vi "init Tests.vi"(8 "error in (no error)":errorcluster caption="Error in", 11 "DeviceInterface Eingang":refnum<class "DeviceInterface.lvclass"> caption="DNL_LabVIEW Object in") -> (0 "error out":errorcluster caption="Error out", 3 "DeviceInterface Ausgang":refnum<class "DeviceInterface.lvclass"> caption="DNL_LabVIEW Object out")   [LabVIEW 2013, in "DeviceInterface.lvclass"]
doc: "Initilisiert die Standard-Tests für das Entsprechende Gerät"
uses:
  DeviceInterface.lvclass
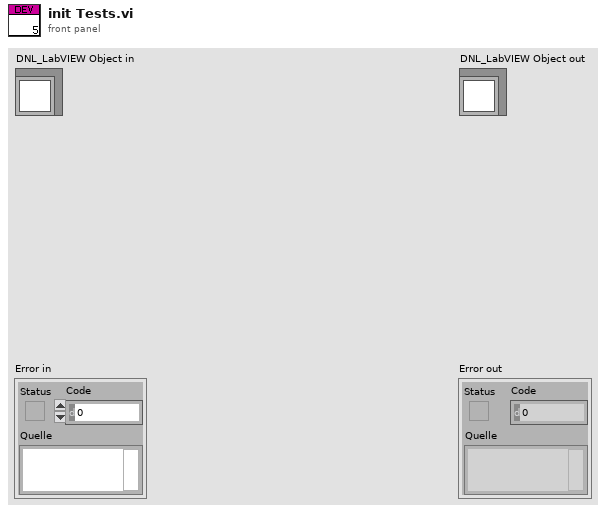
[diagram p1: front panel]
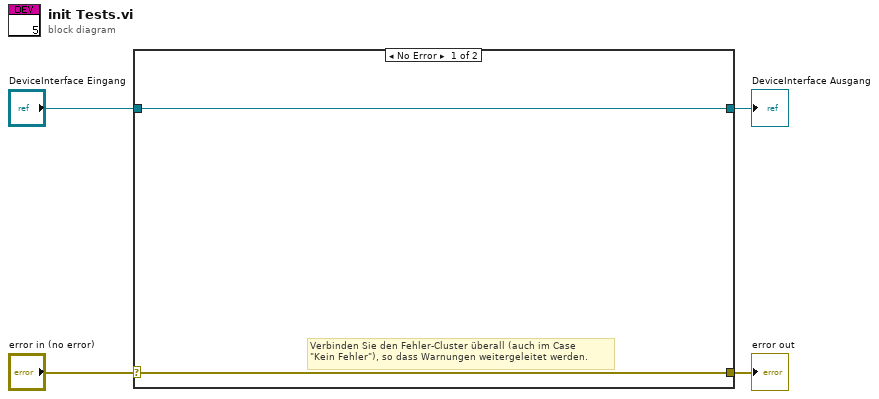
[diagram p0: block diagram]
diagram:
  n1 = case shown="No Error" "error in (no error)" {
    selector: "error in (no error)" -> [w5 w8]
    tunnel: [w5 w8] -> w3
    tunnel: [w6 w7] -> w1
    tunnel: "DeviceInterface Eingang" -> [w6 w7]
    frame No Error {
      # "Verbinden Sie den Fehler-Cluster überall (auch im Case\n\"Kein Fehler\"), so dass Warnungen weitergeleitet werden."
    }
    frame Error {
    }
  }
  "error out" <- w3
  "DeviceInterface Ausgang" <- w1
